vi "SQL查询 (子VI).vi"(8 "错误输入（无错误）":errorcluster, 9 "table输入":string(combo), 10 "condition":string, 11 "columns":string[](array[string])) -> (0 "错误输出":errorcluster, 3 "data":string[][](table))   [LabVIEW 2016]
uses:
  <vilib>/Utility/sysdir.llb/System Directory Type.ctl
  <vilib>/addons/database/Connection.llb/DB Tools Open Connec (String).vi
  <vilib>/addons/database/_DB Variant To Data/Database Variant To Data.xnode
  <vilib>/addons/database/NI_Database_API.lvlib
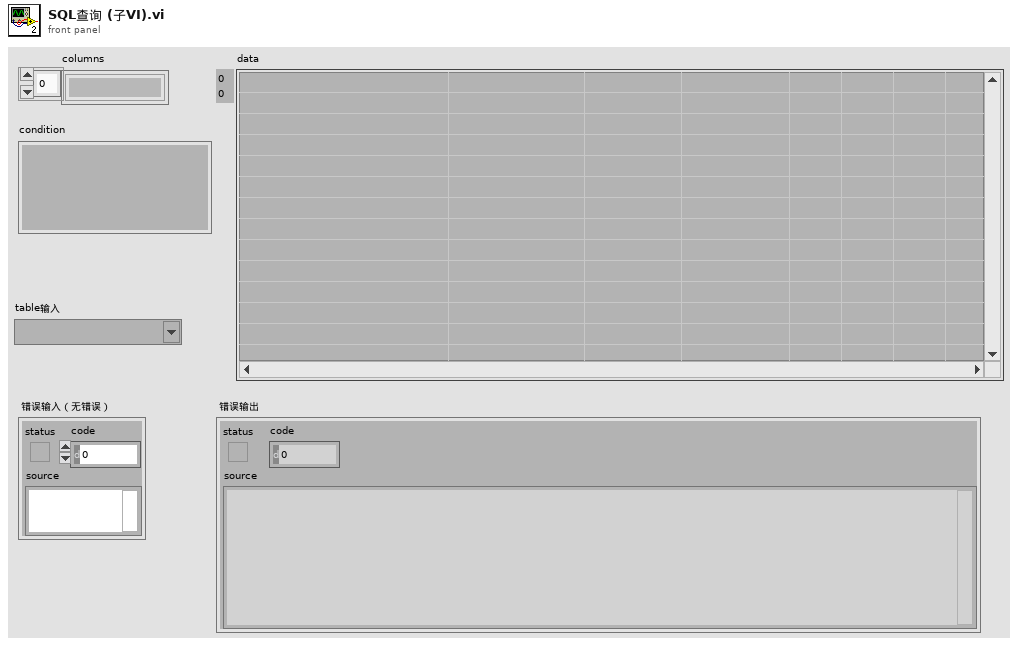
[diagram p1: front panel]
types:
  T1 = typedef "System Directory Type.ctl" = i32
  T2 = typedef "NI_Database_API.lvlib/Conn ObjectReference.ctl" = refnum<k1>
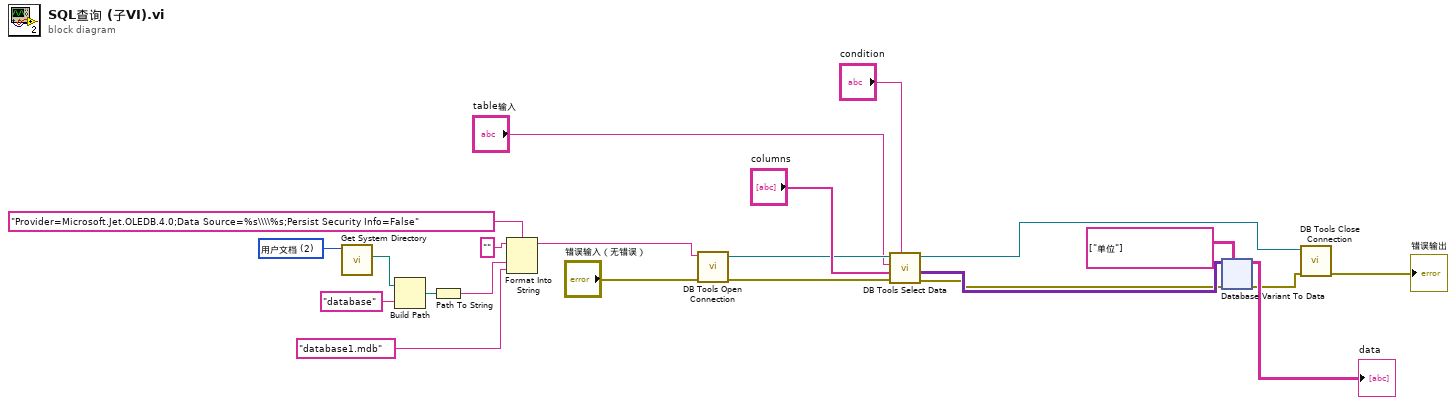
[diagram p0: block diagram]
diagram:
  w2 = T1 2 items=["用户目录"=0, "用户桌面"=1, "用户文档"=2, "用户应用程序数据"=3, "用户设置"=4, "用户临时目录"=5, "公共文档"=6, "公共应用程序数据"=7, "公共设置"=8, "公共缓存"=13, "系统核心库"=9, "系统安装库"=10, "应用程序文件"=11, "启动盘根目录"=12] ("system directory type")
  n1 = call <vilib>:"Get System Directory.vi"("system directory type"=w2) -> ("system directory"=w3:path)  [unwired: 10 in]
  n2 = Build Path(base path=w3, name or relative path="database" ("condition")) -> (appended path=w1:path)
  n3 = Path To String(path=w1) -> (string=w7:string)
  n4 = Format Into String(format string="Provider=Microsoft.Jet.OLEDB.4.0;Data Source=%s\\\\%s;Persist Security Info=False" ("格式字符串"), initial string="" ("初始字符串"), w7, "database1.mdb" ("condition")) -> (resulting string=w10:string)  [unwired: 1 in, 1 out]
  n5 = call-poly <vilib>:"DB Tools Open Connection.vi"("error in (no error)"="错误输入（无错误）", "connection information"=w10) -> ("error out"=w13:errorcluster, "connection reference"=w12:T2)  [unwired: 6 in]
  n6 = call <vilib>:"DB Tools Select Data.vi"("condition"="condition", "error in (no error)"=w13, "columns"="columns", "table"="table输入", "connection reference"=w12) -> ("error out"=w17:errorcluster, "data"=w18:variant[][], "connection reference out"=w20:T2)  [unwired: 1 in]
  n7 = xnode "Database Variant To Data"("database variant"=w18, "error in (no error)"=w17, "type"=string[][] [["单位"]]) -> ("data"=→"data":string[][], "error out"=w21:errorcluster)
  n8 = call <vilib>:"DB Tools Close Connection.vi"("error in (no error)"=w21, "connection reference"=w20) -> ("error out"=→"错误输出":errorcluster)  [unwired: 5 in]
